vi "testConvertToKeyValuePair.vi"(8 "error in (no error)":errorcluster) -> (0 "error out":errorcluster)   [LabVIEW 2018]
doc: "Test the convertToKeyValuePair.vi."
uses:
  src/Utility/keyValuePair/convertToKeyValuePair_double.vi
  <vilib>/addons/_JKI Toolkits/Caraya/classes/Assert/Assert Equal Value_Variant.vi
  src/Utility/keyValuePair/convertToKeyValuePair_integer32bit.vi
  src/Utility/keyValuePair/convertToKeyValuePair_boolean.vi
  src/Utility/keyValuePair/convertToKeyValuePair_string.vi
  src/Utility/keyValuePair/convertToKeyValuePair_1Ddouble.vi
  src/Utility/keyValuePair/convertToKeyValuePair_2Ddouble.vi
  src/Utility/keyValuePair/convertToKeyValuePair_unsignedInteger32bit.vi
  src/Utility/keyValuePair/convertToKeyValuePair_integer64bit.vi
  src/Utility/keyValuePair/convertToKeyValuePair_unsignedInteger64bit.vi
  src/Utility/keyValuePair/convertToKeyValuePair_1Dstring.vi
  <vilib>/addons/_JKI Toolkits/Caraya/classes/Test/Test.lvclass
  <vilib>/addons/_JKI Toolkits/Caraya/classes/Assert/Assert.lvclass
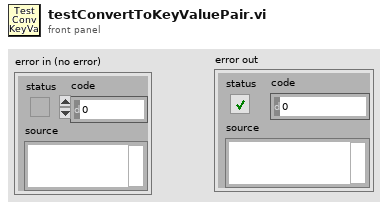
[diagram p1: front panel]
types:
  T1 = cluster{"name":string, "value":dbl[][], "precision (0)":u8}[]
  T2 = cluster{"name":string, "value":dbl[], "precision (0)":u8}[]
  T3 = cluster{"name":string, "value":dbl, "precision (0)":u8}[]
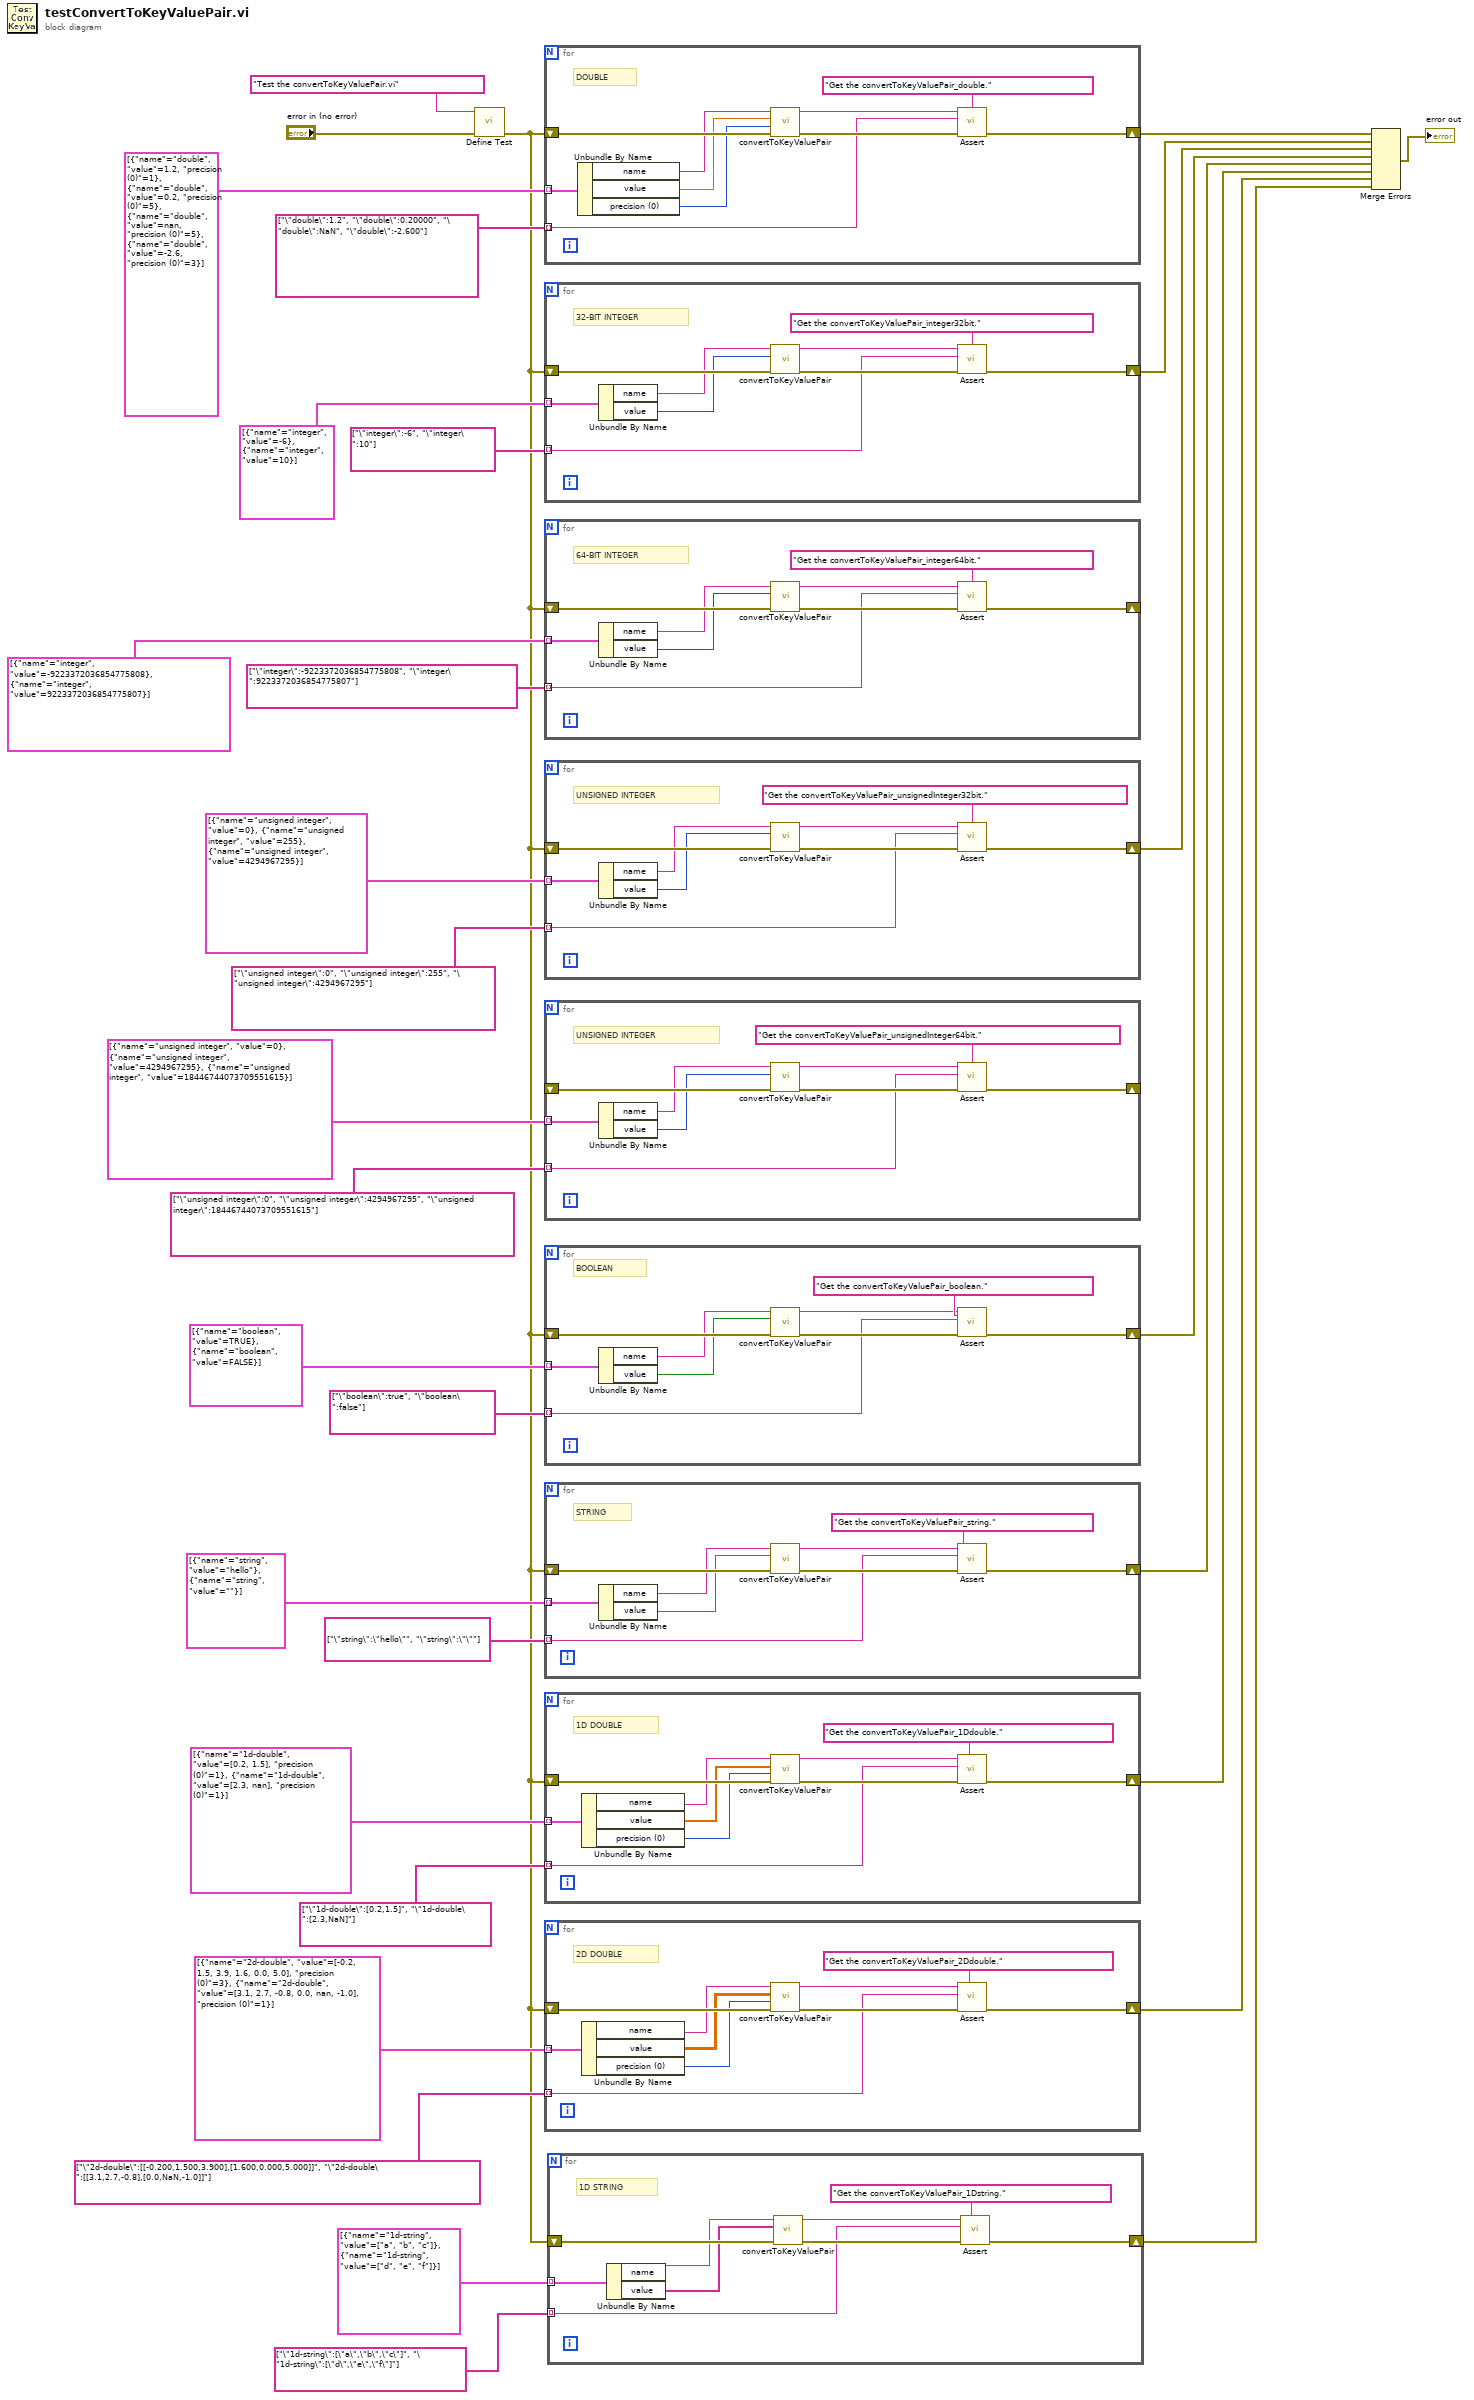
[diagram p0: block diagram]
diagram:
  n1 = call <vilib>:"Define Test.vi"("error in (no error)"="error in (no error)", "Label (VI Title)"="Test the convertToKeyValuePair.vi") -> ("error out"=w2:errorcluster)  [unwired: 9 in]
  n2 = for {
    shift-right: [w42] -> w30
    shift-left: w2 -> [w40]
    tunnel: T3 [{"name"="double", "value"=1.2, "precision (0)"=1}, {"name"="double", "value"=0.2, "precision (0)"=5}, {"name"="double", "value"=nan, "precision (0)"=5}, {"name"="double", "value"=-2.6, "precision (0)"=3}] -> [w38] mode=indexing
    tunnel: string[] ["\"double\":1.2", "\"double\":0.20000", "\"double\":NaN", "\"double\":-2.600"] ("name") -> [w33] mode=indexing
    # "DOUBLE"
    n3 = Unbundle By Name(w38) -> ("name"=w37:string, "value"=w36:dbl, "precision (0)"=w35:u8)
    n4 = call-poly "convertToKeyValuePair.vi"("error in (no error)"=w40, "precision (0)"=w35, "value"=w36, "name"=w37) -> ("error out"=w41:errorcluster, "string converted"=w34:string)  [unwired: 6 in]
    n5 = call-poly <vilib>:"Assert.vi"("Label"="Get the convertToKeyValuePair_double.", "error in (no error)"=w41, "Y"=w33, "X"=w34) -> ("error out"=w42:errorcluster)  [unwired: 7 in]
  }
  n6 = for {
    shift-right: [w51] -> w24
    shift-left: w2 -> [w49]
    tunnel: cluster{"name":string, "value":i32}[] [{"name"="integer", "value"=-6}, {"name"="integer", "value"=10}] -> [w47] mode=indexing
    tunnel: string[] ["\"integer\":-6", "\"integer\":10"] -> [w43] mode=indexing
    # "32-BIT INTEGER"
    n7 = Unbundle By Name(w47) -> ("name"=w46:string, "value"=w45:i32)
    n8 = call-poly "convertToKeyValuePair.vi"("error in (no error)"=w49, "value"=w45, "name"=w46) -> ("error out"=w50:errorcluster, "string converted"=w44:string)  [unwired: 7 in]
    n9 = call-poly <vilib>:"Assert.vi"("Label"="Get the convertToKeyValuePair_integer32bit.", "error in (no error)"=w50, "Y"=w43, "X"=w44) -> ("error out"=w51:errorcluster)  [unwired: 7 in]
  }
  n10 = for {
    shift-right: [w60] -> _
    shift-left: w2 -> [w58]
    tunnel: cluster{"name":string, "value":i64}[] [{"name"="integer", "value"=-9223372036854775808}, {"name"="integer", "value"=9223372036854775807}] -> [w56] mode=indexing
    tunnel: string[] ["\"integer\":-9223372036854775808", "\"integer\":9223372036854775807"] -> [w52] mode=indexing
    # "64-BIT INTEGER"
    n11 = Unbundle By Name(w56) -> ("name"=w55:string, "value"=w54:i64)
    n12 = call-poly "convertToKeyValuePair.vi"("error in (no error)"=w58, "value"=w54, "name"=w55) -> ("error out"=w59:errorcluster, "string converted"=w53:string)  [unwired: 7 in]
    n13 = call-poly <vilib>:"Assert.vi"("Label"="Get the convertToKeyValuePair_integer64bit.", "error in (no error)"=w59, "Y"=w52, "X"=w53) -> ("error out"=w60:errorcluster)  [unwired: 7 in]
  }
  n14 = for {
    shift-right: [w69] -> w10
    shift-left: w2 -> [w67]
    tunnel: cluster{"name":string, "value":u32}[] [{"name"="unsigned integer", "value"=0}, {"name"="unsigned integer", "value"=255}, {"name"="unsigned integer", "value"=4294967295}] -> [w65] mode=indexing
    tunnel: string[] ["\"unsigned integer\":0", "\"unsigned integer\":255", "\"unsigned integer\":4294967295"] -> [w61] mode=indexing
    # "UNSIGNED INTEGER"
    n15 = Unbundle By Name(w65) -> ("name"=w64:string, "value"=w63:u32)
    n16 = call-poly "convertToKeyValuePair.vi"("error in (no error)"=w67, "value"=w63, "name"=w64) -> ("error out"=w68:errorcluster, "string converted"=w62:string)  [unwired: 7 in]
    n17 = call-poly <vilib>:"Assert.vi"("Label"="Get the convertToKeyValuePair_unsignedInteger32bit.", "error in (no error)"=w68, "Y"=w61, "X"=w62) -> ("error out"=w69:errorcluster)  [unwired: 7 in]
  }
  n18 = for {
    shift-right: [w78] -> _
    shift-left: _ -> [w76]
    tunnel: cluster{"name":string, "value":u64}[] [{"name"="unsigned integer", "value"=0}, {"name"="unsigned integer", "value"=4294967295}, {"name"="unsigned integer", "value"=18446744073709551615}] -> [w74] mode=indexing
    tunnel: string[] ["\"unsigned integer\":0", "\"unsigned integer\":4294967295", "\"unsigned integer\":18446744073709551615"] -> [w70] mode=indexing
    # "UNSIGNED INTEGER"
    n19 = Unbundle By Name(w74) -> ("name"=w73:string, "value"=w72:u64)
    n20 = call-poly "convertToKeyValuePair.vi"("error in (no error)"=w76, "value"=w72, "name"=w73) -> ("error out"=w77:errorcluster, "string converted"=w71:string)  [unwired: 7 in]
    n21 = call-poly <vilib>:"Assert.vi"("Label"="Get the convertToKeyValuePair_unsignedInteger64bit.", "error in (no error)"=w77, "Y"=w70, "X"=w71) -> ("error out"=w78:errorcluster)  [unwired: 7 in]
  }
  n22 = for {
    shift-right: [w87] -> w9
    shift-left: w2 -> [w85]
    tunnel: cluster{"name":string, "value":bool}[] [{"name"="boolean", "value"=TRUE}, {"name"="boolean", "value"=FALSE}] -> [w83] mode=indexing
    tunnel: string[] ["\"boolean\":true", "\"boolean\":false"] -> [w79] mode=indexing
    # "BOOLEAN"
    n23 = Unbundle By Name(w83) -> ("name"=w82:string, "value"=w81:bool)
    n24 = call-poly "convertToKeyValuePair.vi"("error in (no error)"=w85, "value"=w81, "name"=w82) -> ("error out"=w86:errorcluster, "string converted"=w80:string)  [unwired: 7 in]
    n25 = call-poly <vilib>:"Assert.vi"("Label"="Get the convertToKeyValuePair_boolean.", "error in (no error)"=w86, "Y"=w79, "X"=w80) -> ("error out"=w87:errorcluster)  [unwired: 7 in]
  }
  n26 = for {
    shift-right: [w96] -> w11
    shift-left: w2 -> [w94]
    tunnel: cluster{"name":string, "value":string}[] [{"name"="string", "value"="hello"}, {"name"="string", "value"=""}] -> [w91] mode=indexing
    tunnel: string[] ["\"string\":\"hello\"", "\"string\":\"\""] -> [w88] mode=indexing
    # "STRING"
    n27 = Unbundle By Name(w91) -> ("name"=w90:string, "value"=w89:string)
    n28 = call-poly "convertToKeyValuePair.vi"("error in (no error)"=w94, "value"=w89, "name"=w90) -> ("error out"=w95:errorcluster, "string converted"=w92:string)  [unwired: 7 in]
    n29 = call-poly <vilib>:"Assert.vi"("Label"="Get the convertToKeyValuePair_string.", "error in (no error)"=w95, "Y"=w88, "X"=w92) -> ("error out"=w96:errorcluster)  [unwired: 7 in]
  }
  n30 = for {
    shift-right: [w106] -> w12
    shift-left: w2 -> [w104]
    tunnel: string[] ["\"1d-double\":[0.2,1.5]", "\"1d-double\":[2.3,NaN]"] -> [w101] mode=indexing
    tunnel: T2 [{"name"="1d-double", "value"=[0.2, 1.5], "precision (0)"=1}, {"name"="1d-double", "value"=[2.3, nan], "precision (0)"=1}] -> [w100] mode=indexing
    # "1D DOUBLE"
    n31 = Unbundle By Name(w100) -> ("name"=w99:string, "value"=w98:dbl[], "precision (0)"=w97:u8)
    n32 = call-poly "convertToKeyValuePair.vi"("error in (no error)"=w104, "presicion (0)"=w97, "value"=w98, "name"=w99) -> ("error out"=w105:errorcluster, "string converted"=w102:string)  [unwired: 6 in]
    n33 = call-poly <vilib>:"Assert.vi"("Label"="Get the convertToKeyValuePair_1Ddouble.", "error in (no error)"=w105, "Y"=w101, "X"=w102) -> ("error out"=w106:errorcluster)  [unwired: 7 in]
  }
  n34 = for {
    shift-right: [w116] -> w13
    shift-left: w2 -> [w114]
    tunnel: string[] ["\"2d-double\":[[-0.200,1.500,3.900],[1.600,0.000,5.000]]", "\"2d-double\":[[3.1,2.7,-0.8],[0.0,NaN,-1.0]]"] -> [w111] mode=indexing
    tunnel: T1 [{"name"="2d-double", "value"=[[-0.2, 1.5, 3.9], [1.6, 0.0, 5.0]], "precision (0)"=3}, {"name"="2d-double", "value"=[[3.1, 2.7, -0.8], [0.0, nan, -1.0]], "precision (0)"=1}] -> [w110] mode=indexing
    # "2D DOUBLE"
    n35 = Unbundle By Name(w110) -> ("name"=w109:string, "value"=w108:dbl[][], "precision (0)"=w107:u8)
    n36 = call-poly "convertToKeyValuePair.vi"("error in (no error)"=w114, "presicion (0)"=w107, "value"=w108, "name"=w109) -> ("error out"=w115:errorcluster, "string converted"=w112:string)  [unwired: 6 in]
    n37 = call-poly <vilib>:"Assert.vi"("Label"="Get the convertToKeyValuePair_2Ddouble.", "error in (no error)"=w115, "Y"=w111, "X"=w112) -> ("error out"=w116:errorcluster)  [unwired: 7 in]
  }
  n38 = for {
    shift-right: [w125] -> w1
    shift-left: w2 -> [w123]
    tunnel: cluster{"name":string, "value":string[]}[] [{"name"="1d-string", "value"=["a", "b", "c"]}, {"name"="1d-string", "value"=["d", "e", "f"]}] -> [w121] mode=indexing
    tunnel: string[] ["\"1d-string\":[\"a\",\"b\",\"c\"]", "\"1d-string\":[\"d\",\"e\",\"f\"]"] -> [w118] mode=indexing
    # "1D STRING"
    n39 = Unbundle By Name(w121) -> ("name"=w120:string, "value"=w119:string[])
    n40 = call-poly "convertToKeyValuePair.vi"("error in (no error)"=w123, "value"=w119, "name"=w120) -> ("error out"=w124:errorcluster, "string converted"=w117:string)  [unwired: 7 in]
    n41 = call-poly <vilib>:"Assert.vi"("Label"="Get the convertToKeyValuePair_1Dstring.", "error in (no error)"=w124, "Y"=w118, "X"=w117) -> ("error out"=w125:errorcluster)  [unwired: 7 in]
  }
  n42 = Merge Errors(w30, w24, w10, w9, w11, w12, w13, w1) -> (→"error out":errorcluster)
